vi "Test Flash.vi"(8 "error in (no error)":errorcluster, 11 "VGC in":refnum<class "PL Inficon VGC.lvclass">) -> (0 "error out":errorcluster, 1 "checksum":u32, 2 "error word":u16, 3 "VGC out":refnum<class "PL Inficon VGC.lvclass">)   [LabVIEW 2015, in "PL Inficon VGC.lvclass"]
doc: "Tests flash."
uses:
  PL Inficon VGC.lvclass
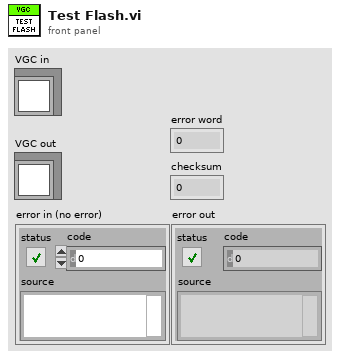
[diagram p1: front panel]
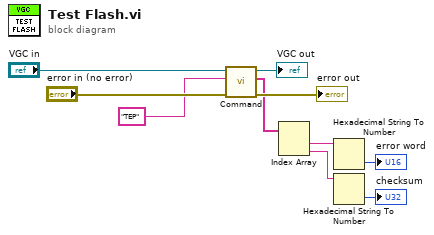
[diagram p0: block diagram]
diagram:
  n1 = call "Command.vi"("error in (no error)"="error in (no error)", "command"="TEP", "VGC in"="VGC in") -> ("error out"=→"error out":errorcluster, "response data"=w5:string[], "VGC out"=→"VGC out":refnum<class "PL Inficon VGC.lvclass">)  [unwired: 6 in]
  n2 = Index Array(array=w5) -> (element #1=w4:string, element #2=w1:string)  [unwired: 2 in]
  n3 = Hexadecimal String To Number(string=w4) -> (number=→"error word":u32)  [unwired: 2 in, 1 out]
  n4 = Hexadecimal String To Number(string=w1) -> (number=→"checksum":u32)  [unwired: 2 in, 1 out]
